vi "oa_FIR Preprocess Filter Order Estimation.vi"(7 "filter types":T2(ring), 8 "error in (no error)":errorcluster, 9 "fs [Hz]":dbl=1.0, 10 "ripple specs [dB]":cluster{"pass band":dbl, "stop band":dbl}={"pass band"=0.1, "stop band"=60.0} {"stop band" format="%0.2f"; "pass band" format="%0.2f"}, 11 "freq specs [Hz]":T1={"fpass 1"=0.125, "fstop 1"=0.45, "fpass 2"=0.125, "fstop 2"=0.45} {"fstop 2" format="%0.2f"; "fpass 2" format="%.3f"; "fstop 1" format="%0.2f"; "fpass 1" format="%.3f"}) -> (0 "error out":errorcluster, 1 "low cutoff freq: fl":dbl, 2 "high cutoff freq: fh":dbl, 3 "estimated order":i32, 4 "beta":dbl)   [LabVIEW 2017, in "SoundVib_RefDataProcess.lvlib"]
uses:
  <vilib>/addons/Sound and Vibration/Order Analysis/Referece Data Processing/SoundVib_RefDataProcess.lvlib
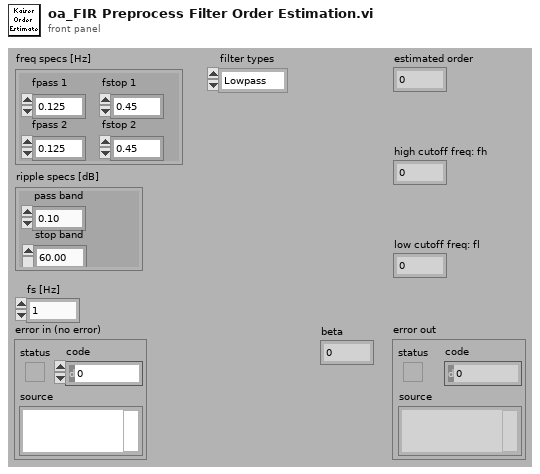
[diagram p1: front panel]
types:
  T1 = cluster{"fpass 1":dbl, "fstop 1":dbl, "fpass 2":dbl, "fstop 2":dbl}
  T2 = enum32{"Lowpass", "Highpass", "Bandpass", "Bandstop"}
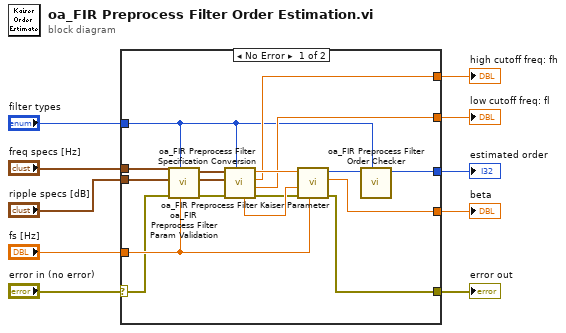
[diagram p0: block diagram]
diagram:
  n1 = case shown="No Error" "error in (no error)" {
    selector: "error in (no error)" -> [w14 w28]
    tunnel: "freq specs [Hz]" -> [w27 _]
    tunnel: "ripple specs [dB]" -> [w26 _]
    tunnel: "filter types" -> [w12 _]
    tunnel: [w11 _] -> w7
    tunnel: [w21 _] -> w6
    tunnel: [w20 _] -> w5
    tunnel: "fs [Hz]" -> [w19 _]
    tunnel: [w18 _] -> w3
    tunnel: [w15 w28] -> w1
    frame No Error {
      n2 = call <vilib>:"oa_FIR Preprocess Filter Param Validation.vi"("fs [Hz]"=w19, "filter types"=w12, "error in (no error)"=w14, "ripple specs [dB]"=w26, "freq specs [Hz]"=w27) -> ("error out"=w17:errorcluster, "dup ripple specs [dB]"=w24:cluster{"pass band":dbl, "stop band":dbl}, "dup freq specs [Hz]"=w25:T1)  [unwired: 4 in]
      n3 = call <vilib>:"oa_FIR Preprocess Filter Specification Conversion.vi"("filter types"=w12, "error in"=w17, "ripple specs [dB]"=w24, "freq specs"=w25) -> ("error out"=w16:errorcluster, "low cutoff freq: fl"=w20:dbl, "high cutoff freq: fh"=w21:dbl, "min transition band"=w23:dbl, "A stop (dB)"=w22:dbl)  [unwired: 3 in]
      n4 = call <vilib>:"oa_FIR Preprocess Filter Kaiser Parameter.vi"("fs [Hz]"=w19, "error in (no error)"=w16, "A stop"=w22, "delta f [Hz]"=w23) -> ("error out"=w15:errorcluster, "beta"=w18:dbl, "estimated order"=w13:i32)  [unwired: 5 in]
      n5 = call <vilib>:"oa_FIR Preprocess Filter Order Checker.vi"("filter types"=w12, "order in"=w13) -> ("order out"=w11:i32)  [unwired: 9 in]
    }
    frame Error {
    }
  }
  "estimated order" <- w7
  "high cutoff freq: fh" <- w6
  "low cutoff freq: fl" <- w5
  "beta" <- w3
  "error out" <- w1
